vi "New.vi"(7 "Velocity direction in":cluster{"X":dbl, "Y":dbl}, 10 "Flying saucer in":refnum<class "Flying Saucer.lvclass">) -> (3 "Missile out":refnum<class "Missile.lvclass">)   [LabVIEW 2024, in "Missile.lvclass"]
doc: "MIT Licence\nCopyright (c) 2024 David Grollier"
uses:
  Missile.lvclass
  Flying Saucer/Flying Saucer.lvclass
  Movable.lvclass/Movable.ctl
  Game Board Component.lvclass/Game Board Component.ctl
  Game Componants.lvclass/Game Componants.ctl
  Missile.lvclass/Missile.ctl
  Movable.lvclass
  Game Board Component.lvclass
  Game Componants.lvclass
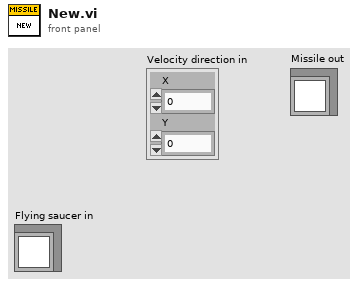
[diagram p1: front panel]
types:
  T1 = typedef "Coordinates.ctl" = cluster{"x":dbl, "y":dbl}
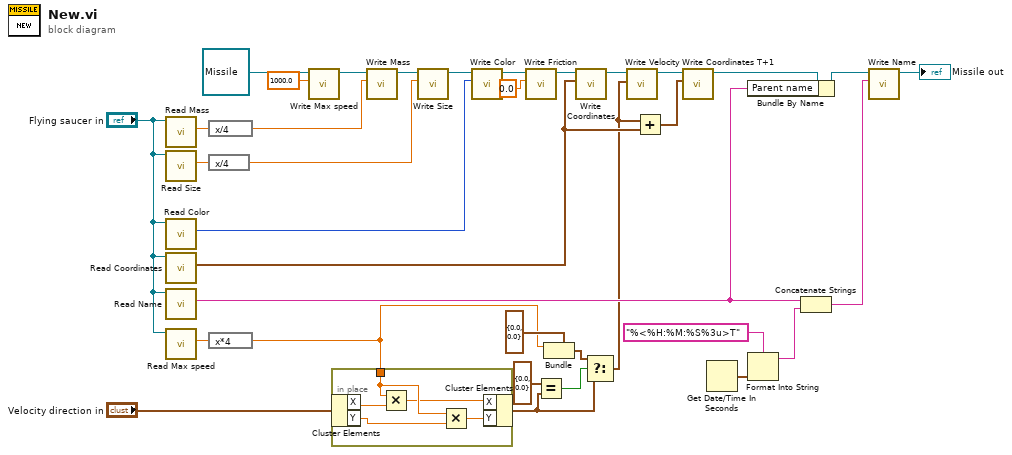
[diagram p0: block diagram]
diagram:
  n1 = call "Read Mass.vi"("Movable in"="Flying saucer in") -> ("Mass"=w26:dbl)  [unwired: 10 in]
  n2 = call "Read Size.vi"("Movable in"="Flying saucer in") -> ("Size"=w28:dbl)  [unwired: 10 in]
  n3 = call "Read Color.vi"("Game Board Component in"="Flying saucer in") -> ("color"=w30:u32)  [unwired: 10 in]
  n4 = call "Read Coordinates.vi"("Game Componants in"="Flying saucer in") -> ("Coordinates"=w13:T1)  [unwired: 10 in]
  n5 = call "Read Name.vi"("Game Board Component in"="Flying saucer in") -> ("Name"=w18:string)  [unwired: 10 in]
  n6 = call "Read Max speed.vi"("Movable in"="Flying saucer in") -> ("Max speed"=w29:dbl)  [unwired: 10 in]
  n7 = expression code="x/4"(w26) -> (w25:dbl)
  n8 = expression code="x/4"(w28) -> (w27:dbl)
  n9 = expression code="x*4"(w29) -> (w5:dbl)
  n10 = call "Write Max speed.vi"("Max speed"=1000.0, "Movable in"=refnum<class "Missile.lvclass"> refnum ("Missile in")) -> ("Movable out"=w24:refnum<class "Missile.lvclass">)  [unwired: 9 in]
  n11 = in-place {
    in-place-border: w5 -> [w38]
    n12 = in-place-cluster #1("Velocity direction in") -> ("X"=w40:dbl, "Y"=w39:dbl)
    n13 = Multiply(x=w38, y=w40) -> (x*y=w37:dbl)
    n14 = Multiply(x=w38, y=w39) -> (x*y=w36:dbl)
    n15 = in-place-cluster #1("X"=w37, "Y"=w36) -> (w2:cluster{"X":dbl, "Y":dbl})
  }
  n16 = call "Write Mass.vi"("Mass"=w25, "Movable in"=w24) -> ("Movable out"=w33:refnum<class "Missile.lvclass">)  [unwired: 9 in]
  n17 = call "Write Size.vi"("Size"=w27, "Movable in"=w33) -> ("Movable out"=w10:refnum<class "Missile.lvclass">)  [unwired: 9 in]
  n18 = call "Write Color.vi"("color"=w30, "Game Board Component in"=w10) -> ("Game Board Component out"=w34:refnum<class "Missile.lvclass">)  [unwired: 9 in]
  n19 = call "Write Friction.vi"("Friction"=0.0, "Movable in"=w34) -> ("Movable out"=w35:refnum<class "Missile.lvclass">)  [unwired: 9 in]
  n20 = Equal?(x=cluster{"X":dbl, "Y":dbl} {"X"=0.0, "Y"=0.0}, y=w2) -> (x = y?=w4:bool)
  n21 = Bundle(cluster=cluster{"X":dbl, "Y":dbl} {"X"=0.0, "Y"=0.0} ("x"), "X"=w5) -> (w3:cluster{"X":dbl, "Y":dbl})  [unwired: 1 in]
  n22 = call "Write Coordinates.vi"("Coordinates"=w13, "Game Componants in"=w35) -> ("Game Componants out"=w9:refnum<class "Missile.lvclass">)  [unwired: 9 in]
  n23 = Select(t=w3, s=w4, f=w2) -> (s? t:f=w1:cluster{"X":dbl, "Y":dbl})
  n24 = call "Write Velocity.vi"("Velocity"=w1, "Movable in"=w9) -> ("Movable out"=w8:refnum<class "Missile.lvclass">)  [unwired: 9 in]
  n25 = Add(x=w1, y=w13) -> (x+y=w12:T1)
  n26 = call "Write Coordinates T+1.vi"("Coordinates"=w12, "Movable in"=w8) -> ("Movable out"=w14:refnum<class "Missile.lvclass">)  [unwired: 9 in]
  n27 = Get Date/Time In Seconds() -> (seconds since 1Jan1904=w19:timestamp)
  n28 = Bundle By Name(cluster=w14, "Parent name"=w18) -> (w22:refnum<class "Missile.lvclass">)
  n29 = Format Into String(format string="%<%H:%M:%S%3u>T", w19) -> (resulting string=w17:string)  [unwired: 2 in, 1 out]
  n30 = Concatenate Strings(w18, w17) -> (w15:string)
  n31 = call "Write Name.vi"("Name"=w15, "Game Board Component in"=w22) -> ("Game Board Component out"=→"Missile out":refnum<class "Missile.lvclass">)  [unwired: 9 in]
